vi "PH_Synchrolock_Watch.PC Get data.vi"(0 "i ref in":refnum<vi>, 5 "error IO":errorcluster) -> (14 "i ref out":refnum<vi>, 19 "error out":errorcluster)   [LabVIEW 2014, in "PH_Synchrolock_Watch.lvlib"]
doc: "This is the proc case \"Get Data\": It communicates with hardware to get data and writes them to own attributes."
uses:
  PH_Synchrolock_Watch.lvlib
  PH_TKTDS-30xx/PH_TKTDS-30xx.Waveform to fetch.ctl
  PH_StatusHandler/PH_StatusHandler.Status.ctl
  PH_TKTDS-30xx/PH_TKTDS-30xx.lvlib
  PH_StatusHandler/PH_StatusHandler.lvlib
panel:
  in  "Waveform to fetch":T1={"Source"="CH1", "Waveform Start"=1, "Waveform End"=10000}
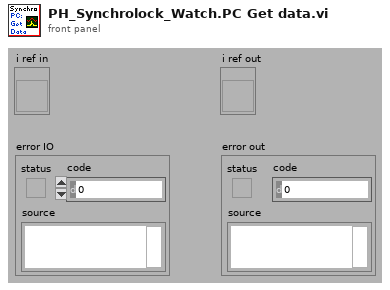
[diagram p1: front panel]
types:
  T1 = typedef "PH_TKTDS-30xx.lvlib/PH_TKTDS-30xx.Waveform to fetch.ctl" = cluster{"Source":string, "Waveform Start":i32, "Waveform End":i32}
  T2 = typedef "PH_StatusHandler.lvlib/PH_StatusHandler.Status.ctl" = i16
  T3 = typedef "PH_Synchrolock_Watch.lvlib/PH_Synchrolock_Watch.i attribute.ctl" = cluster{"GUI Refs":cluster{"Mean Phase Graph":refnum<vi>, "RF Amplitude Graph":refnum<vi>, "Mira Amplitude Graph":refnum<vi>, "MIRA State":refnum<vi>, "Mean Phase":refnum<vi>, "RF Amplitude":refnum<vi>, "Mira Amplitude":refnum<vi>, "Mean Phase in range?":refnum<vi>, "RF Amplitude above limit?":refnum<vi>, "Mira Amplitude in range?":refnum<vi>, "Mean phase upper limit":refnum<vi>, "Mean phase lower limit":refnum<vi>, "RF Amplitude lower limit":refnum<vi>, "Mira Amplitude lower limit":refnum<vi>, "Mira Amplitude upper limit":refnum<vi>, "Waveform End":refnum<vi>, "Mira scope":refnum<vi>, "Reset Mira warning":refnum<vi>}, "Status":cluster{"Reset Warning":bool}, "Mean Phase":cluster{"Current Value":dbl, "Upper Limit":dbl, "Lower Limit":dbl, "Data":cluster{dbl[], dbl[]}}, "RF":cluster{"Current Value":dbl, "Lower Limit":dbl, "Data":cluster{dbl[], dbl[]}}, "MIRA":cluster{"Current Value":dbl, "Upper Limit":dbl, "Lower Limit":dbl, "Data":cluster{dbl[], dbl[]}}, "Waveform End":i32}
  T4 = typedef "PH_TKTDS-30xx.lvlib/PH_TKTDS-30xx.i attribute.ctl" = cluster{"Default VISA Resource":string, "VISA Resource Name":refnum<visa-resource-name>, "Revision":cluster{"Instrument Driver":string, "Instrument Firmware":string}, "Selftest":cluster{"Result":u32, "Message":string}, "Channels":T5[], "Trigger Configuration":T6, "Acquisition Configuration":T7, "Fetched Waveforms":T8[], "GUI Refs":T9, "GUI Refs Channels":refnum<vi>[], "State":T2, "Error Message":string, "Allow Prdc Loop?":bool}
  T5 = typedef "PH_TKTDS-30xx.lvlib/PH_TKTDS-30xx.Channel Config.ctl" = cluster{"Channel Name":string, "Input Impedance":string, "Max Input Frequency":string, "Vertical Coupling":i32, "Channel Enabled":bool, "Probe Attenuation":dbl, "Vertical Range":dbl, "Vertical Offset":dbl}
  T6 = typedef "PH_TKTDS-30xx.lvlib/PH_TKTDS-30xx.Trigger Config.ctl" = cluster{"Source":string, "Slope":i32, "Level [V]":dbl}
  T7 = typedef "PH_TKTDS-30xx.lvlib/PH_TKTDS-30xx.Acquisition Config.ctl" = cluster{"Time base":dbl, "Record Length":u16, "Start Time":dbl, "Type":i32, "Continuous":bool}
  T8 = typedef "PH_TKTDS-30xx.lvlib/PH_TKTDS-30xx.fetched Waveform.ctl" = cluster{"Source":string, "Actual Points":u32, "Initial X":dbl, "X Increment":dbl, "Waveform Array":dbl[]}
  T9 = typedef "PH_TKTDS-30xx.lvlib/PH_TKTDS-30xx.GUI Refs.ctl" = cluster{"Trigger":refnum<vi>, "Acquisition":refnum<vi>, "Graph":refnum<vi>, "State":refnum<vi>, "Delete":refnum<vi>, "Channel to be positioned":refnum<vi>, "Postion":refnum<vi>, "Display Intensity":refnum<vi>, "VISA Resource":refnum<vi>}
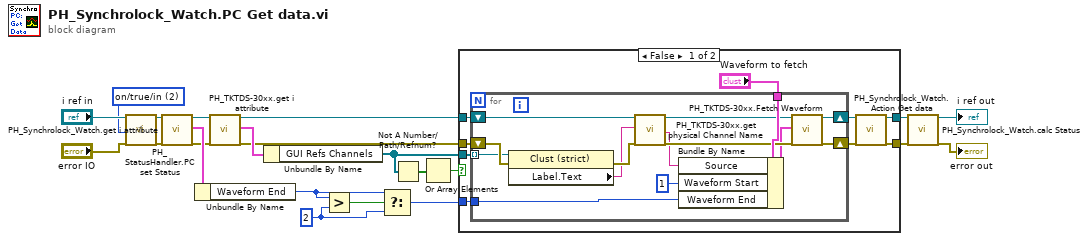
[diagram p0: block diagram]
diagram:
  w1 = T2 2 items=["no info", "off/false/out", "on/true/in", "Failure", "Alarm", "Status 1", "Status 2", "Status 3"] ("Status")
  w4 = 2 ("y")
  n1 = call "PH_StatusHandler.PC set Status.vi"("i ref in"="i ref in", "Status"=w1, "error in (no error)"="error IO") -> ("i ref out"=w17:refnum<vi>, "error out"=w16:errorcluster)  [unwired: 15 in]
  n2 = call "PH_Synchrolock_Watch.get i attribute.vi"("i ref in"=w17, "error in (no error)"=w16) -> ("i ref out"=w15:refnum<vi>, "i attribute"=w19:T3, "error out"=w14:errorcluster)  [unwired: 15 in]
  n3 = Unbundle By Name(w19) -> ("Waveform End"=w3:i32)
  n4 = call "PH_TKTDS-30xx.get i attribute.vi"("i ref in"=w15, "error in (no error)"=w14) -> ("i ref out"=w8:refnum<vi>, "i attribute"=w13:T4, "error out"=w9:errorcluster)  [unwired: 15 in]
  n5 = Unbundle By Name(w13) -> ("GUI Refs Channels"=w10:refnum<vi>[])
  n6 = Greater?(x=w3, y=w4) -> (0:w5:bool)
  n7 = Select(t=w3, s=w5, f=w4) -> (s? t:f=w2:i32)
  n8 = Not A Number/Path/Refnum?(number/path/refnum=w10) -> (NaN/Path/Refnum?=w12:bool[])
  n9 = Or Array Elements(Boolean array=w12) -> (logical OR=w11:bool)
  n10 = case shown="False" w11 {
    tunnel: [w28 w47] -> w7
    tunnel: [w27 w46] -> w6
    tunnel: w10 -> [w26 _]
    tunnel: w8 -> [w25 w47]
    tunnel: w9 -> [w24 w46]
    tunnel: w2 -> [w23 _]
    frame False {
      n11 = for {
        shift-right: [w42] -> w29
        shift-left: w24 -> [w41]
        shift-right: [w43] -> w30
        shift-left: w25 -> [w44]
        tunnel: "Waveform to fetch" -> [w45]
        tunnel: w26 -> [w39] mode=indexing
        tunnel: w23 -> [w32]
        n12 = property class="Clust (strict)"(reference=w39, error in=w41) -> (error out=w40:errorcluster, "Label.Text"=w38:string)  [unwired: 1 out]
        n13 = call "PH_TKTDS-30xx.get physical Channel Name.vi"("i ref in"=w44, "GUI Element Name"=w38, "error in"=w40) -> ("i ref out"=w35:refnum<vi>, "Physical Channel Name"=w33:string, "error out"=w36:errorcluster)  [unwired: 14 in]
        n14 = Bundle By Name(cluster=w45, "Source"=w33, "Waveform Start"=1, "Waveform End"=w32) -> (w34:T1)
        n15 = call "PH_TKTDS-30xx.Fetch Waveform.vi"("i ref in"=w35, "Waveform to fetch"=w34, "error IO"=w36) -> ("i ref out"=w43:refnum<vi>, "error out"=w42:errorcluster)  [unwired: 15 in]
      }
      n16 = call "PH_Synchrolock_Watch.Action Get data.vi"("i ref in"=w30, "error IO"=w29) -> ("i ref out"=w28:refnum<vi>, "error out"=w27:errorcluster)  [unwired: 16 in]
    }
    frame True {
    }
  }
  n17 = call "PH_Synchrolock_Watch.calc Status.vi"("i ref in"=w7, "error in"=w6) -> ("i ref out"=→"i ref out":refnum<vi>, "error out"=→"error out":errorcluster)  [unwired: 16 in]
